vi "Control.vi"() -> ()   [LabVIEW 2010]
uses:
  Fear Conditioning/GlobalFear.vi
panel:
  out "Shock\nPeriod":bool
  in  "Manual Reset":bool
  out "sum":dbl
  out "Shock":bool
  in  "Safety":bool
  in  "Threshold\n(inches)":dbl
  in  "stop 2":bool
  out "Activity monitor":dynamicdata(graph)
  in  "Mouse Axis":bool
  in  "DPI":dbl=350.0
  in  "Activity mouse":refnum<visa-resource-name>
  out "Iteration":dbl
  out "Sound":dbl
  out "Stimulus":dbl
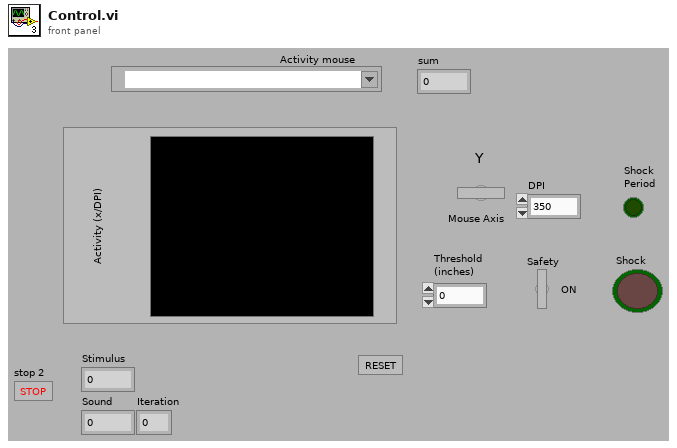
[diagram p1: front panel]
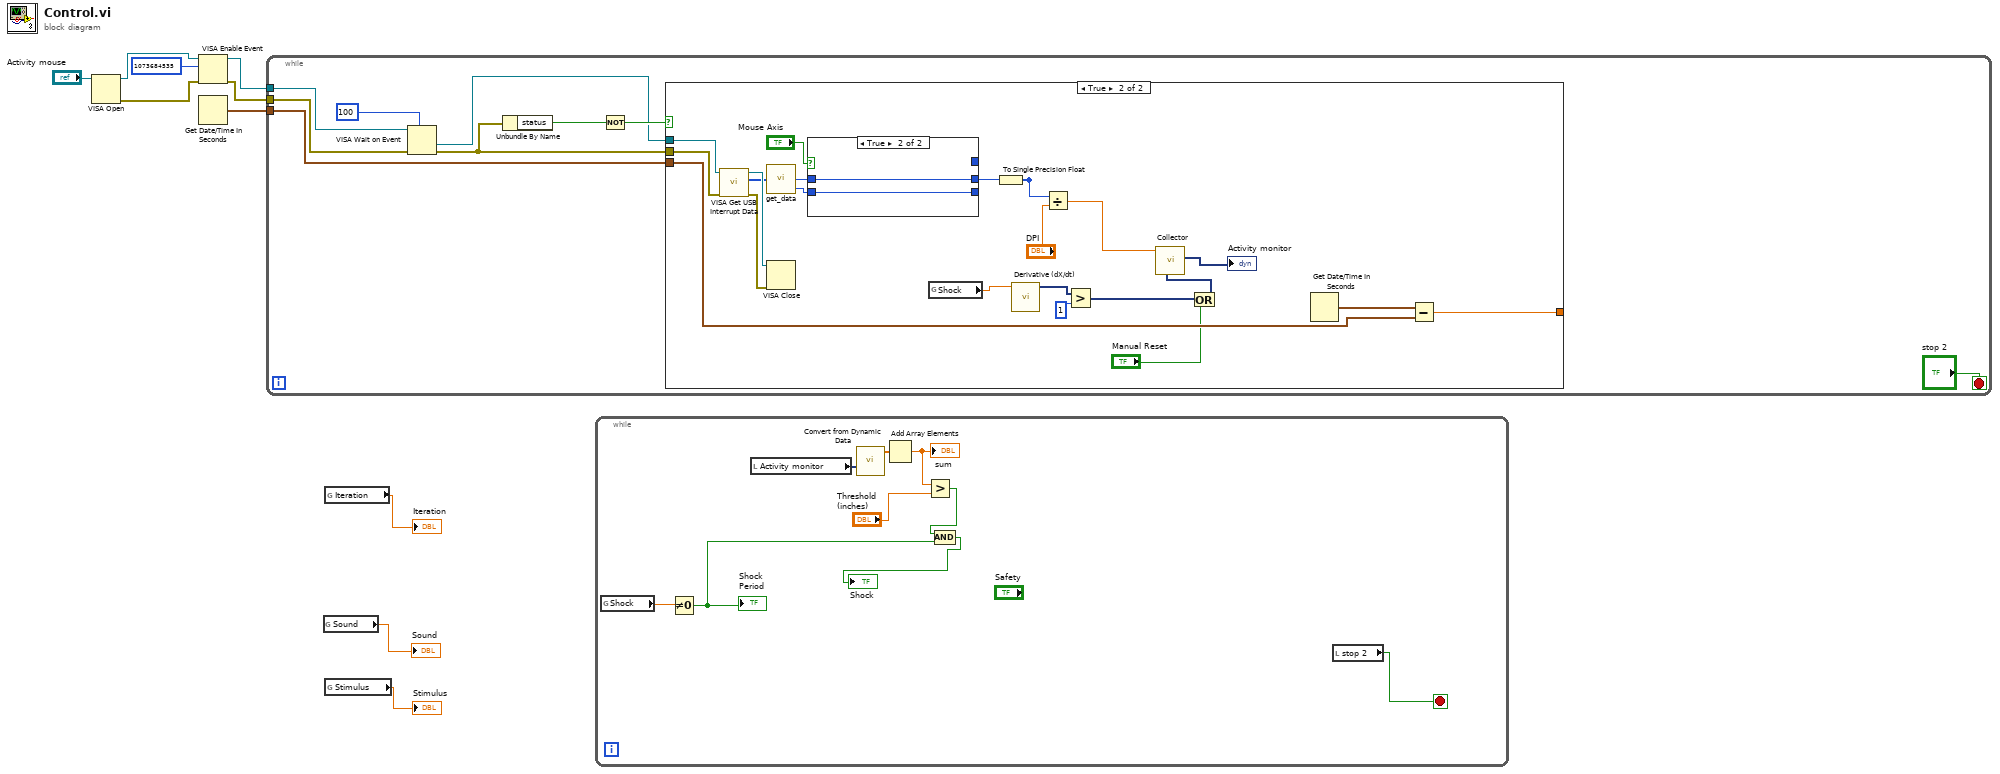
[diagram p0: block diagram]
diagram:
  n1 = VISA Open(VISA resource name="Activity mouse") -> (VISA resource name=w7:refnum<visa-resource-name>, error out=w6:errorcluster)  [unwired: 1 in, 3 out]
  n2 = VISA Enable Event(8:w6, 10:u32 1073684535 ("event type"), 11:w7) -> (0:w3:errorcluster, 3:w4:refnum<visa-resource-name>)  [unwired: 1 out]
  n3 = Get Date/Time In Seconds() -> (seconds since 1Jan1904=w1:timestamp)
  n4 = while {
    tunnel: w4 -> [w19]
    tunnel: w3 -> [w18]
    tunnel: w1 -> [w17]
    stop <- "stop 2" stop-if-true
    n5 = VISA Wait on Event(7:u32 100 ("timeout (0)"), 8:w18, 11:w19) -> (0:w12:errorcluster, 1:w13:refnum<visa-resource-name>)  [unwired: 4 out]
    n6 = Unbundle By Name(w12) -> ("status"=w14:bool)
    n7 = Not(x=w14) -> (.not. x?=w15:bool)
    n8 = case shown="True" w15 {
      tunnel: w13 -> [_ w37]
      tunnel: w12 -> [_ w36]
      tunnel: w17 -> [_ w34]
      tunnel: [_ w33] -> _
      frame False {
      }
      frame True {
        n9 = call <vilib>:"VISA Get USB Interrupt Data.vi"("error in (no error)"=w36, "VISA USB Intr Event"=w37) -> ("error out"=w38:errorcluster, "data buffer"=w35:u8[], "VISA USB Intr Event out"=w39:refnum<visa-resource-name>)  [unwired: 7 out]
        n10 = call "get_data.vi"("data buffer"=w35) -> ("X Value"=w30:i8, "Y Value"=w29:i8)  [unwired: 1 out]
        n11 = VISA Close(VISA resource name=w39, error in (no error)=w38) -> ()  [unwired: 1 out]
        n12 = case shown="True" "Mouse Axis" {
          tunnel: w30 -> [w41 w44]
          tunnel: [w42 w44] -> w28
          tunnel: w29 -> [w42 w43]
          tunnel: [w41 _] -> _
          tunnel: [_ w43] -> _
          frame False {
          }
          frame True {
          }
        }
        n13 = global read "GlobalFear.vi" "Shock"() -> (w25:dbl)
        n14 = To Single Precision Float(number=w28) -> ()  [unwired: 1 out]
        n15 = call "Derivative (dX/dt)"("Signals"=w25) -> ("Result"=w23:dynamicdata)  [unwired: 5 in, 1 out]
        n16 = Divide(x=w28, y="DPI") -> (x/y=w26:dbl)
        n17 = Greater?(x=w23, y=1) -> (0:w22:dynamicdata)
        n18 = Or(x=w22, y="Manual Reset") -> (x .or. y?=w20:dynamicdata)
        n19 = call "Collector"("Reset"=w20, "Signals"=w26) -> ("Collected Signals"=→"Activity monitor":dynamicdata)  [unwired: 8 in, 1 out]
        n20 = Get Date/Time In Seconds() -> (seconds since 1Jan1904=w40:timestamp)
        n21 = Subtract(x=w40, y=w34) -> (x-y=w33:dbl)
      }
    }
  }
  n22 = global read "GlobalFear.vi" "Sound"() -> (→"Sound":dbl)
  n23 = global read "GlobalFear.vi" "Iteration"() -> (→"Iteration":dbl)
  n24 = global read "GlobalFear.vi" "Stimulus"() -> (→"Stimulus":dbl)
  n25 = while {
    stop <- w51 stop-if-true
    n26 = global read "GlobalFear.vi" "Shock"() -> (w48:dbl)
    n27 = Not Equal To 0?(x=w48) -> (x != 0?=w46:bool)
    "Shock\nPeriod" <- w46
    n28 = local read "Activity monitor"() -> (w53:dynamicdata)
    n29 = call "Convert from Dynamic Data"("Dynamic Data Type"=w53) -> ("Array"=w52:dbl[])  [unwired: 3 in]
    n30 = Add Array Elements(numeric array=w52) -> (sum=w50:dbl)
    "sum" <- w50
    n31 = Greater?(x=w50, y="Threshold\n(inches)") -> (0:w47:bool)
    n32 = And(x=w47, y=w46) -> (x .and. y?=→"Shock":bool)
    n33 = local read "stop 2"() -> (w51:bool)
  }
